vi "Wavelet Cluster.vi"(3 "Cluster":T1) -> ()   [LabVIEW 2014]
panel:
  in  "Wavelet Family":string(combo)
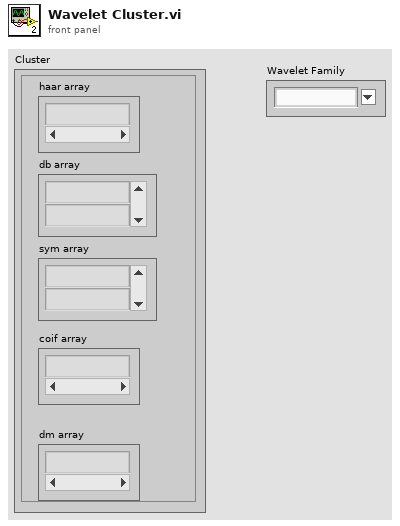
[diagram p1: front panel]
types:
  T1 = cluster{"haar array":string[], "db array":string[], "sym array":string[], "coif array":string[], "dm array":string[]}
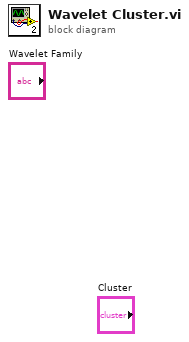
[diagram p0: block diagram]
diagram:
